vi "ModbusTest.vi"() -> ()   [LabVIEW 2016]
uses:
  <vilib>/NI Modbus.llb/MB Serial Master Query Write Multiple Registers (poly).vi
  <vilib>/NI Modbus.llb/MB Serial Master Query Read Holding Registers (poly).vi
  <vilib>/NI Modbus.llb/MB Serial Master Query Write Multiple Coils (poly).vi
  <vilib>/NI Modbus.llb/MB Serial Master Query Read Coils (poly).vi
panel:
  out "number":u32
  in  "Registers":u16[](array[numeric])
  in  "Coils in":bool[](array[boolean])=[TRUE, FALSE, TRUE]
  out "Coils out":bool[](array[boolean])
  out "Exception Code":u8 format="%.0x"
  out "error out":errorcluster
  out "Input Registers":u16[](array[numeric])
  in  "error in (no error)":errorcluster
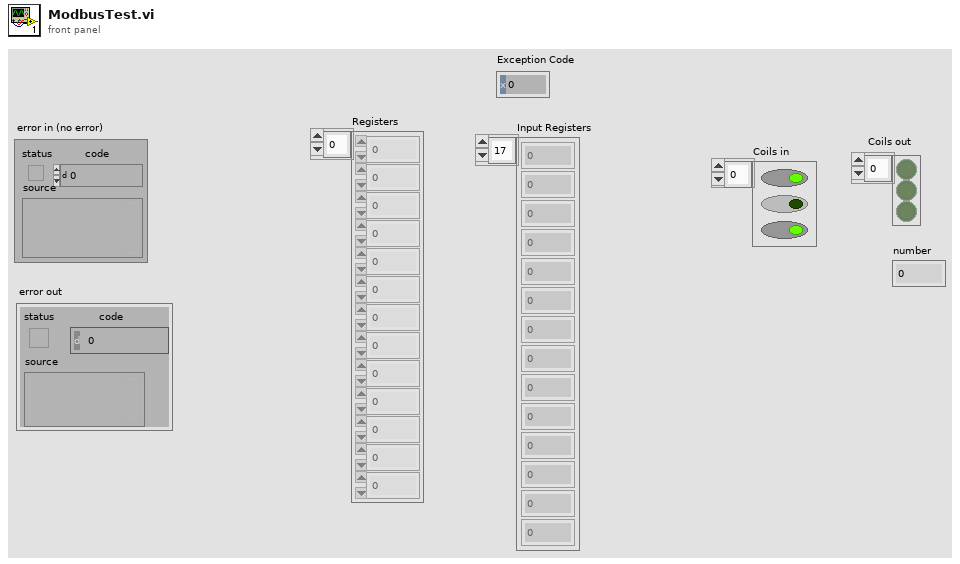
[diagram p1: front panel]
types:
  T1 = cluster{"Mode":enum16{"RTU", "ASCII"}, "Slave Address":u8}
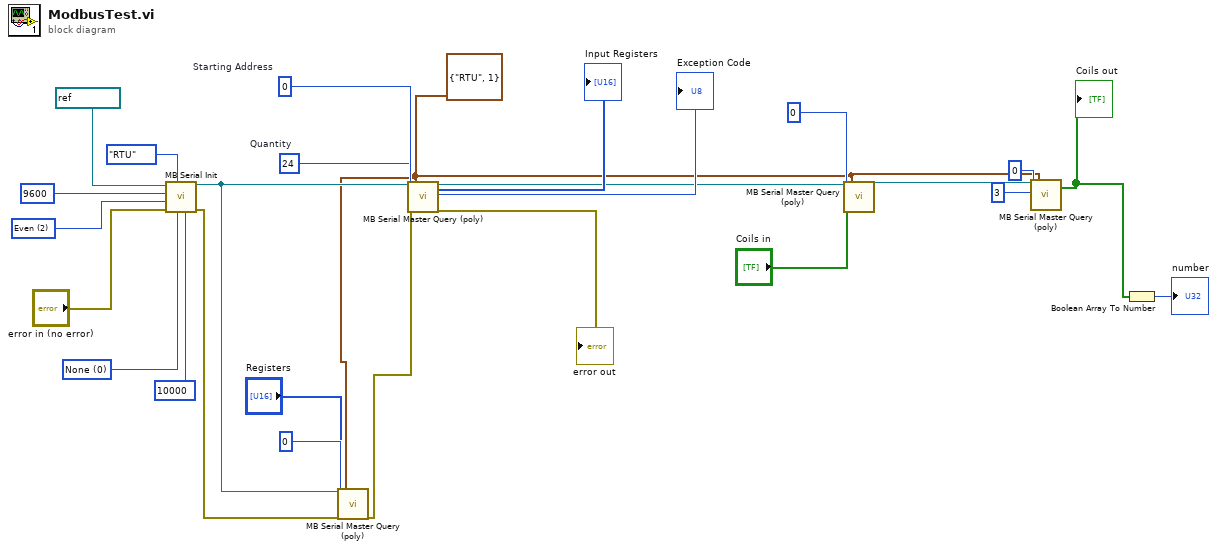
[diagram p0: block diagram]
diagram:
  w6 = T1 {"Mode"=enum."RTU", "Slave Address"=1} ("Serial Parameters")
  w18 = u16 24  # Quantity
  w19 = u16 0  # Starting Address
  w21 = u16 0 items=["None", "XON/XOFF", "RTS/CTS", "XON/XOFF & RTS/CTS", "DTR/DSR", "XON/XOFF & DTR/DSR"] ("Flow Control")
  w24 = u16 2 items=["None", "Odd", "Even", "Mark", "Space"] ("Parity")
  n1 = call <vilib>:"MB Serial Init.vi"("Timeout"=u32 10000, "Flow Control"=w21, "Mode"=enum16{"RTU", "ASCII"}."RTU", "error in (no error)"="error in (no error)", "Parity"=w24, "Baud Rate"=u32 9600, "VISA resource name"=refnum<visa-resource-name> "COM4") -> ("error out"=w8:errorcluster, "VISA resource name out"=w9:refnum<visa-resource-name>)  [unwired: 3 in]
  n2 = call-poly <vilib>:"MB Serial Master Query (poly).vi"("VISA resource name"=w9, "Starting Address"=u16 0, "Registers"="Registers", "error in"=w8, "Serial Parameters"=w6) -> ("error out"=w7:errorcluster)  [unwired: 12 in, 2 out]
  n3 = call-poly <vilib>:"MB Serial Master Query (poly).vi"("VISA resource name"=w9, "Starting Address"=w19, "Quantity"=w18, "error in"=w7, "Serial Parameters"=w6) -> ("VISA resource name out"=w14:refnum<visa-resource-name>, "Holding Registers"=→"Input Registers":u16[], "Exception Code"=→"Exception Code":u8, "error out"=→"error out":errorcluster)  [unwired: 11 in]
  n4 = call-poly <vilib>:"MB Serial Master Query (poly).vi"("VISA resource name"=w14, "Starting Address"=u16 0, "Coils"="Coils in", "Serial Parameters"=w6) -> ("VISA resource name out"=w3:refnum<visa-resource-name>)  [unwired: 13 in, 2 out]
  n5 = call-poly <vilib>:"MB Serial Master Query (poly).vi"("VISA resource name"=w3, "Starting Address"=u16 0, "Quantity"=u16 3, "Serial Parameters"=w6) -> ("Coils"=w2:bool[])  [unwired: 12 in, 3 out]
  "Coils out" <- w2
  n6 = Boolean Array To Number(Boolean array=w2) -> (number=→"number":u32)
